vi "Move Motors.vi"(0 "Current Motor Position past home (um)":string, 5 "XY Mouse Position":string, 7 "pix/micron":dbl, 9 "Camera Resolution X":i64, 11 "Camera Resolution Y":i64) -> (4 "Motor XY After Moving":string)   [LabVIEW 2014]
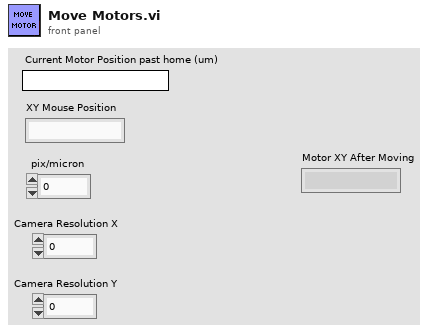
[diagram p1: front panel]
types:
  T1 = enum16{"Default", "Set Statuses", "Set Parameters", "Save Parameter"}
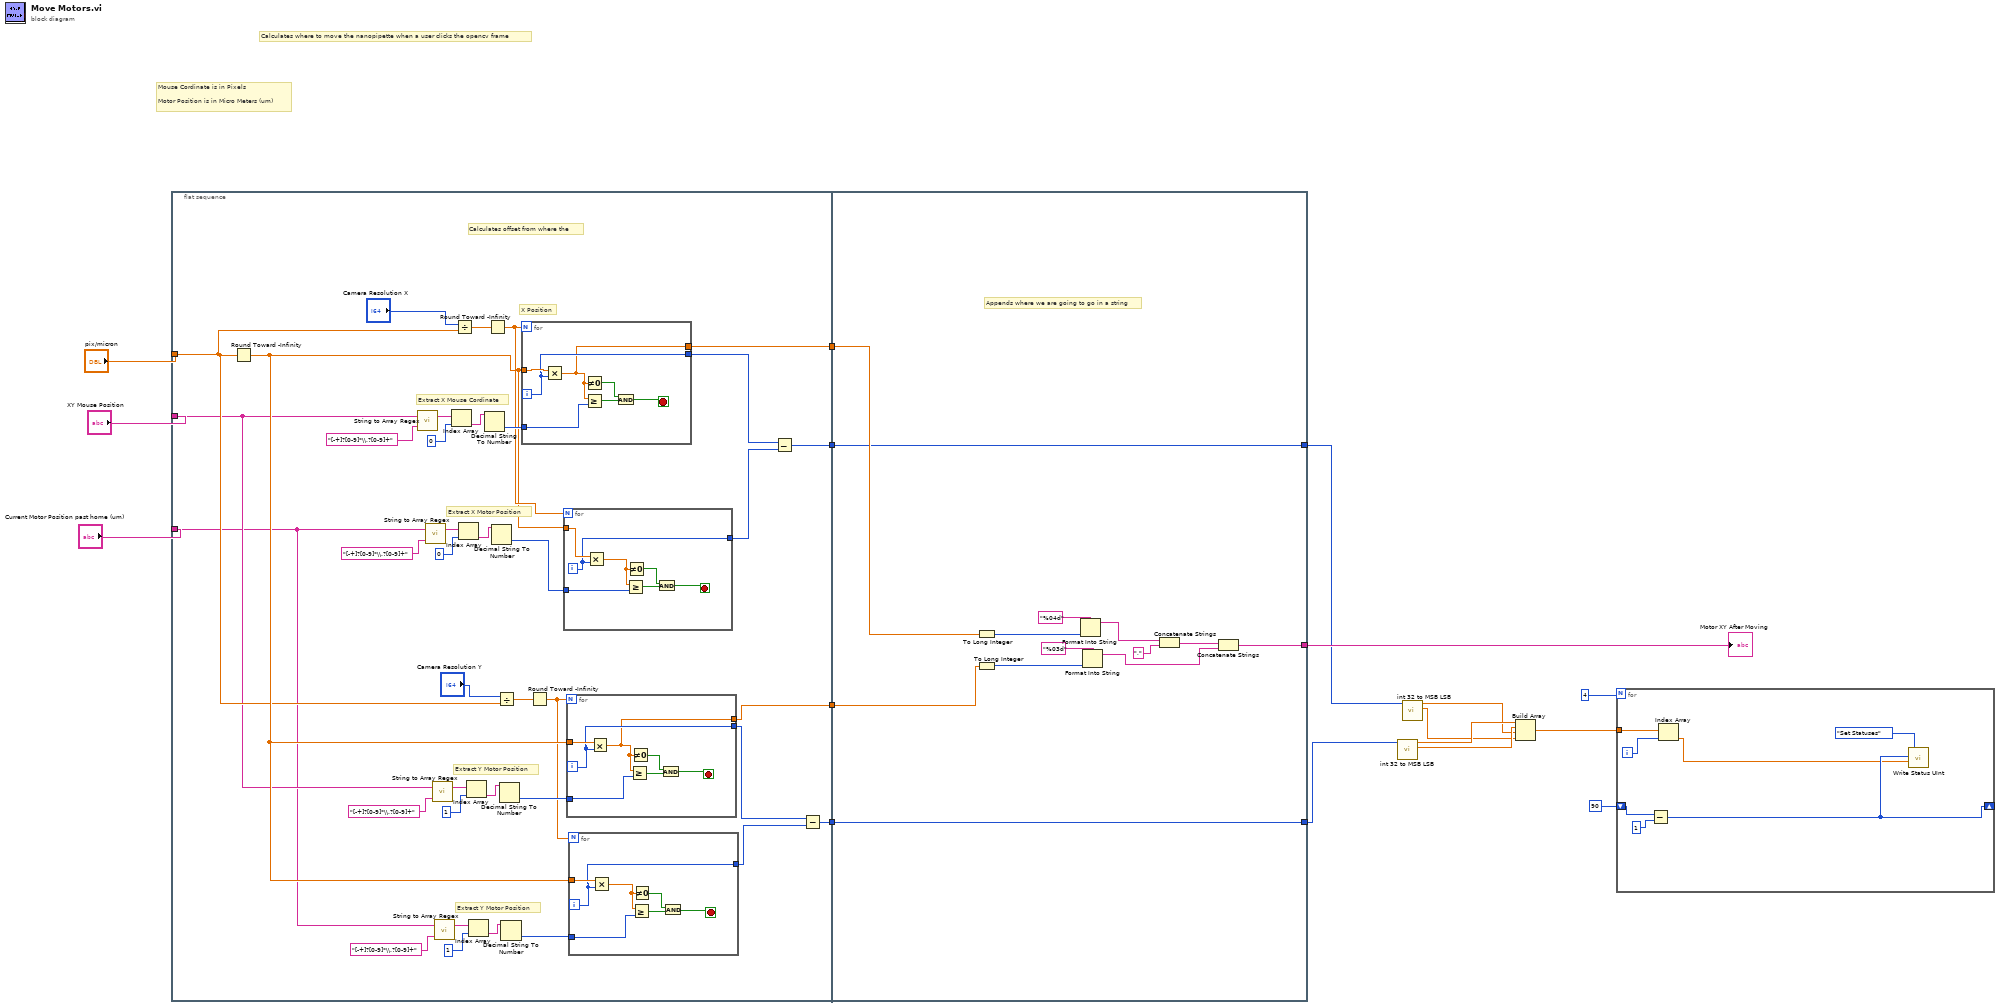
[diagram p0: block diagram]
diagram:
  # "Calculates where to move the nanopipette when a user clicks the opencv frame"
  # "Mouse Cordinate is in Pixels\n\nMotor Position is in Micro Meters (um)"
  n1 = flat-sequence {
    tunnel: "pix/micron" -> [w26]
    tunnel: "XY Mouse Position" -> [w21]
    tunnel: "Current Motor Position past home (um)" -> [w20]
    tunnel: [w40] -> w14
    tunnel: [w22] -> w13
    tunnel: [w19] -> w12
    tunnel: [w18] -> w11
    tunnel: [w86] -> w10
    tunnel: w11 -> [w85]
    tunnel: w12 -> [w84]
    tunnel: w13 -> [w87]
    tunnel: w14 -> [w88]
    tunnel: [w85] -> w9
    tunnel: [w84] -> w8
    frame #0 {
      # "Calculates offset from where the"
      # "Extract Y Motor Position"
      # "Extract Y Motor Position"
      # "Extract X Motor Position"
      # "Extract X Mouse Cordinate"
      # "X Position"
      n2 = Round Toward -Infinity(1:w26) -> (0:w29:dbl)
      n3 = call "String to Array Regex.vi"("Regex"="[-+]?[0-9]*\\.?[0-9]+", "Message"=w21) -> ("String to Array"=w52:string[])  [unwired: 1 in]
      n4 = call "String to Array Regex.vi"("Regex"="[-+]?[0-9]*\\.?[0-9]+", "Message"=w20) -> ("String to Array"=w48:string[])  [unwired: 1 in]
      n5 = call "String to Array Regex.vi"("Regex"="[-+]?[0-9]*\\.?[0-9]+", "Message"=w21) -> ("String to Array"=w39:string[])  [unwired: 1 in]
      n6 = call "String to Array Regex.vi"("Regex"="[-+]?[0-9]*\\.?[0-9]+", "Message"=w20) -> ("String to Array"=w34:string[])  [unwired: 1 in]
      n7 = Index Array(array=w52, index=0) -> (element=w49:string)
      n8 = Divide(x="Camera Resolution X", y=w26) -> (x/y=w54:dbl)
      n9 = Index Array(array=w48, index=0) -> (element=w46:string)
      n10 = Index Array(array=w39, index=1) -> (element=w37:string)
      n11 = Index Array(array=w34, index=1) -> (element=w32:string)
      n12 = Decimal String To Number(string=w49) -> (number=w50:i32)  [unwired: 2 in, 1 out]
      n13 = Round Toward -Infinity(1:w54) -> (0:w44:dbl)
      n14 = Decimal String To Number(string=w46) -> (number=w42:i32)  [unwired: 2 in, 1 out]
      n15 = Divide(x="Camera Resolution Y", y=w26) -> (x/y=w28:dbl)
      n16 = Decimal String To Number(string=w37) -> (number=w35:i32)  [unwired: 2 in, 1 out]
      n17 = Decimal String To Number(string=w32) -> (number=w30:i32)  [unwired: 2 in, 1 out]
      n18 = for {
        N: w44 -> [_]
        tunnel: w50 -> [w83]
        tunnel: w29 -> [w80]
        tunnel: [w78] -> w41
        tunnel: [w77] -> w40
        i -> [w78]
        stop <- w79 stop-if-true
        n19 = Multiply(x=w80, y=w78) -> (x*y=w77:dbl)
        n20 = Greater Or Equal?(x=w77, y=w83) -> (x >= y?=w82:bool)
        n21 = Not Equal To 0?(x=w77) -> (x != 0?=w81:bool)
        n22 = And(x=w81, y=w82) -> (x .and. y?=w79:bool)
      }
      n23 = Round Toward -Infinity(1:w28) -> (0:w25:dbl)
      n24 = for {
        N: w44 -> [_]
        tunnel: w29 -> [w73]
        tunnel: [w71] -> w43
        tunnel: w42 -> [w70]
        i -> [w71]
        stop <- w74 stop-if-true
        n25 = Multiply(x=w73, y=w71) -> (x*y=w72:dbl)
        n26 = Greater Or Equal?(x=w72, y=w70) -> (x >= y?=w76:bool)
        n27 = Not Equal To 0?(x=w72) -> (x != 0?=w75:bool)
        n28 = And(x=w75, y=w76) -> (x .and. y?=w74:bool)
      }
      n29 = for {
        N: w25 -> [_]
        tunnel: w35 -> [w69]
        tunnel: w29 -> [w66]
        tunnel: [w64] -> w23
        tunnel: [w63] -> w22
        i -> [w64]
        stop <- w65 stop-if-true
        n30 = Multiply(x=w66, y=w64) -> (x*y=w63:dbl)
        n31 = Greater Or Equal?(x=w63, y=w69) -> (x >= y?=w68:bool)
        n32 = Not Equal To 0?(x=w63) -> (x != 0?=w67:bool)
        n33 = And(x=w67, y=w68) -> (x .and. y?=w65:bool)
      }
      n34 = for {
        N: w25 -> [_]
        tunnel: w30 -> [w62]
        tunnel: w29 -> [w59]
        tunnel: [w57] -> w24
        i -> [w57]
        stop <- w58 stop-if-true
        n35 = Multiply(x=w59, y=w57) -> (x*y=w56:dbl)
        n36 = Greater Or Equal?(x=w56, y=w62) -> (x >= y?=w61:bool)
        n37 = Not Equal To 0?(x=w56) -> (x != 0?=w60:bool)
        n38 = And(x=w60, y=w61) -> (x .and. y?=w58:bool)
      }
      n39 = Subtract(x=w41, y=w43) -> (x-y=w19:i32)
      n40 = Subtract(x=w23, y=w24) -> (x-y=w18:i32)
    }
    frame #1 {
      # "Appends where we are going to go in a string"
      n41 = To Long Integer(number=w88) -> (32bit integer=w90:i32)
      n42 = To Long Integer(number=w87) -> (32bit integer=w92:i32)
      n43 = Format Into String(format string="%04d", w90) -> (resulting string=w93:string)  [unwired: 2 in, 1 out]
      n44 = Format Into String(format string="%03d", w92) -> (resulting string=w96:string)  [unwired: 2 in, 1 out]
      n45 = Concatenate Strings(w93, ",") -> (w94:string)
      n46 = Concatenate Strings(w94, w96) -> (w86:string)
    }
  }
  n47 = call "int 32 to MSB LSB.vi"("Signed 32 Bit Int"=w9) -> ("LSB NUM"=w3:dbl, "MSB NUM"=w4:dbl)  [unwired: 9 in]
  n48 = call "int 32 to MSB LSB.vi"("Signed 32 Bit Int"=w8) -> ("LSB NUM"=w1:dbl, "MSB NUM"=w2:dbl)  [unwired: 9 in]
  n49 = Build Array(w4, w3, w2, w1) -> (w7:dbl[])
  n50 = for {
    N: 4 -> [_]
    tunnel: w7 -> [w99]
    shift-right: [w101] -> _
    shift-left: 90 -> [w102]
    i -> [w98]
    n51 = Subtract(x=w102, y=1) -> (x-y=w101:i32)
    n52 = Index Array(array=w99, index=w98) -> (element=w97:dbl)
    n53 = call "Write Status UInt.vi"("Status Value"=w97, "Status Number"=w101, "Command"=T1."Set Statuses") -> ()  [unwired: 4 in, 1 out]
  }
  "Motor XY After Moving" <- w10
